vi "Main_define_mosaic.vi"(0 "ROI manager":refnum<vi>, 1 "XY positions IN":dbl[][](array[numeric]), 2 "queue ASI stage":refnum<queue>, 5 "ROI manager":i32(listbox), 7 "Start acquisition":bool, 9 "XY positions":refnum<vi>, 11 "error in":errorcluster, 12 "Mosaic size X":i32(ring) items=["1", "3", "5"], 13 "Mosaic size Y":i32(ring) items=["1", "3", "5"], 14 "FOV size (um)":dbl=200.0 min=0.0 step=0.1 format="%#.1f") -> (3 "XY positions OUT":dbl[][](array[numeric]), 4 "Next task":T1, 10 "XY graph":cluster{dbl[], dbl[]}[](array[cluster]), 15 "error out":errorcluster)   [LabVIEW 2015]
uses:
  CONTROLS/Q_ASI_stage_element.ctl
  CONTROLS/Q_main_element.ctl
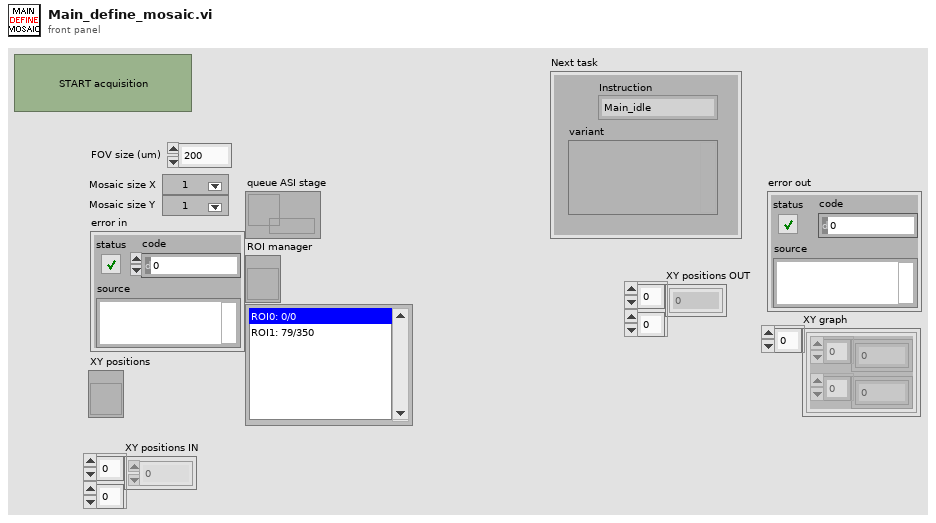
[diagram p1: front panel]
types:
  T1 = typedef "Q_main_element.ctl" = cluster{"variant":variant, "Instruction":enum16{"Main_idle", "Main_initialize", "Main_initialize_TDMS", "Main_initialize_Queue", "Main_error", "Main_DAQ_initialization_results", "Main_ASI_initialization_results", "Main_Piezo_initialization_results", "Main_Valve_initialization_results", "Main_Pump_initialization_results", "Main_CAMERA_initialization_results", "Main_FPGA_initialization_results", "Main_DAQ_error", "Main_ASI_error", "Main_Piezo_error", "Main_CAMERA_error", "Main_Valve_error", "Main_Pump_error", "Main_FPGA_error", "Main_start_acquiring", "Main_not_acquiring", "Main_acquiring", "Main_stop_acquiring", "Main_change_exposure", "Main_change_z_scan_parameters", "Main_define_ROI", "Main_define_mosaic", "Main_read_kinetic_time", "Main_cooler", "Main_read_temperature", "Main_save_XY", "Main_load_XY", "Main_discard_XY", "Main_move_to_XY", "Main_measure_QPD", "Main_autofocus_calibration", "Main_autofocus_initialization", "Main_autofocus_stop", "Main_save_PID", "Main_change_H_valve_position", "Main_two_way_valve", "Main_save_movie", "Main_init_single_scan", "Main_single_scan", "Main_stop_single_scan", "Main_merFISH_illumination_parameters", "Main_merFISH_buffer_probe_list", "Main_merFISH_injections_procedure", "Main_merFISH_save_setpoint", "Main_merFISH_DAPI_parameters", "Main_merFISH_Brightfield_parameters", "Main_merFISH_save_embryo_ROI", "Main_merFISH_init", "Main_merFISH_resume", "Main_merFISH_start_autofocus", "Main_merFISH_open_close_valve_merFISH", "Main_merFISH_open_close_valve_photobleaching", "Main_merFISH_hybridization", "Main_merFISH_move_to_ROI", "Main_merFISH_wait_stabilization", "Main_merFISH_move_to_REF", "Main_merFISH_scan", "Main_merFISH_photobleaching_injection", "Main_merFISH_photobleaching", "Main_merFISH_send_email", "Main_merFISH_close", "Main_STOP"}}
  T2 = typedef "Q_ASI_stage_element.ctl" = cluster{"variant":variant, "Instruction":enum16{"ASI_idle", "ASI_initialize", "ASI_error", "ASI_security_stop", "ASI_read_XYZ", "ASI_up", "ASI_down", "ASI_left", "ASI_right", "ASI_save_XY", "ASI_move_to_XY", "ASI_brightfield", "ASI_init_scan", "ASI_init_merFISH", "ASI_move_to_XY_merFISH", "ASI_move_to_Z_merFISH", "ASI_init_autofocus_search_merFISH", "ASI_close_autofocus_search_merFISH", "ASI_adjust_piezo_autofocus_merFISH", "ASI_set_piezo_autofocus_to_reference_position_merFISH_TL", "ASI_close_merFISH", "ASI_stop"}}
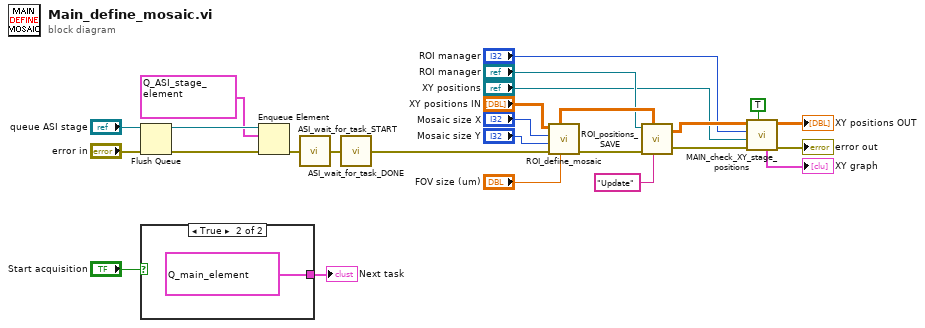
[diagram p0: block diagram]
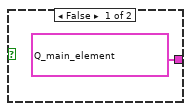
[diagram p2: hidden frame]
diagram:
  n1 = Flush Queue(queue="queue ASI stage", error in (no error)="error in") -> (queue out=w20:refnum<queue>, error out=w23:errorcluster)  [unwired: 1 out]
  n2 = case shown="True" "Start acquisition" {
    tunnel: [T1 {"variant"=variant, "Instruction"=enum."Main_not_acquiring"} ("Q_main_element") T1 {"variant"=variant, "Instruction"=enum."Main_acquiring"} ("Q_main_element")] -> w2
    frame False {
    }
    frame True {
    }
  }
  "Next task" <- w2
  n3 = Enqueue Element(queue=w20, element=T2 {"variant"=variant, "Instruction"=enum."ASI_save_XY"}, error in (no error)=w23) -> (error out=w18:errorcluster)  [unwired: 1 in, 2 out]
  n4 = call "ASI_wait_for_task_START.vi"("error in"=w18) -> ("error out"=w17:errorcluster)
  n5 = call "ASI_wait_for_task_DONE.vi"("error in"=w17) -> ("error out"=w16:errorcluster)
  n6 = call "ROI_define_mosaic.vi"("FOV size (um)"="FOV size (um)", "error in"=w16, "Mosaic size Y"="Mosaic size Y", "Mosaic size X"="Mosaic size X", "XY positions IN"="XY positions IN") -> ("error out"=w13:errorcluster, "XY positions OUT"=w14:dbl[][])  [unwired: 3 in]
  n7 = call "ROI_positions_SAVE.vi"("Choice"="Update", "XY positions"=w14, "error in"=w13, "ROI LstBox Refnum"="ROI manager") -> ("error out"=w10:errorcluster, "XY positions OUT"=w9:dbl[][])  [unwired: 2 in]
  n8 = call "MAIN_check_XY_stage_positions.vi"("Update display properties?"=TRUE, "error in"=w10, 7:"XY positions"="XY positions", "ROI manager"="ROI manager", 9:"XY positions"=w9) -> ("error out"=→"error out":errorcluster, "XY positions OUT"=→"XY positions OUT":dbl[][], "XY graph"=→"XY graph":cluster{dbl[], dbl[]}[])  [unwired: 1 in, 1 out]
